vi "Facade.vi"(0 "Data In":T4, 2 "Display State In":T2, 3 "Container State":T3) -> (6 "Data Out":T4, 7 "Display State Out":T2, 8 "Action":T1)   [LabVIEW 2015, in "Vowel.xctl"]
uses:
  Vowel.xctl
  Vowel.Properties.ctl
  <vilib>/_xctls/Container State.ctl
  State.ctl
  <vilib>/_xctls/Action.ctl
  <vilib>/_xctls/XControlSupport.lvlib
panel:
  in  "Level is":enum16{"total power", "per component"}(ring)
  in  "Frequency (Hz)":string
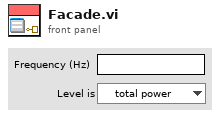
[diagram p1: front panel]
types:
  T1 = typedef "XControlSupport.lvlib/Action.ctl" = cluster{"Data Changed?":bool, "State Changed?":bool, "Action Name":string}
  T2 = typedef "Vowel.xctl/State.ctl" = cluster{"enable menu":bool, "ctls":cluster{"Freq":refnum<vi>, "Phase":refnum<vi>}}
  T3 = typedef "XControlSupport.lvlib/Container State.ctl" = cluster{"Indicator?":bool, "Run Mode?":bool, " Refnum":refnum<vi>}
  T4 = typedef "Vowel.xctl/Vowel.Properties.ctl" = cluster{"Freqs":string, "Set level":enum16{"Total", "Per component"}, "Freq":dbl[], "weights":dbl[]}
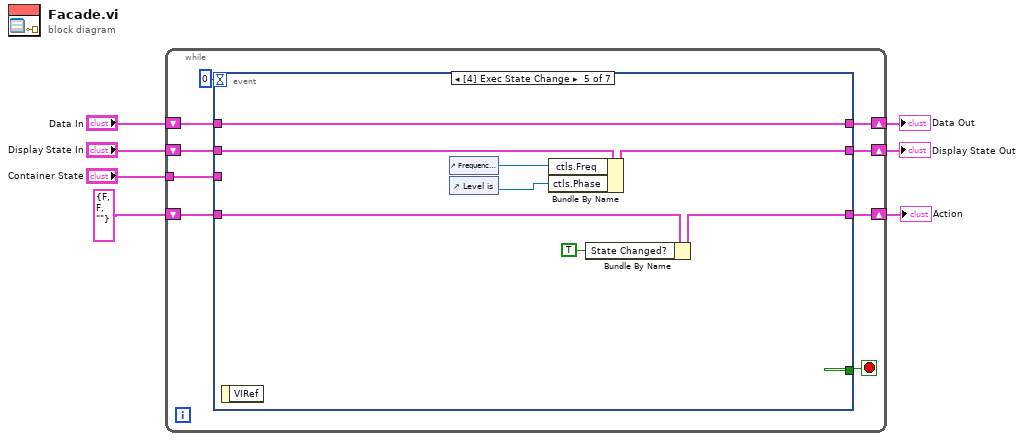
[diagram p0: block diagram]
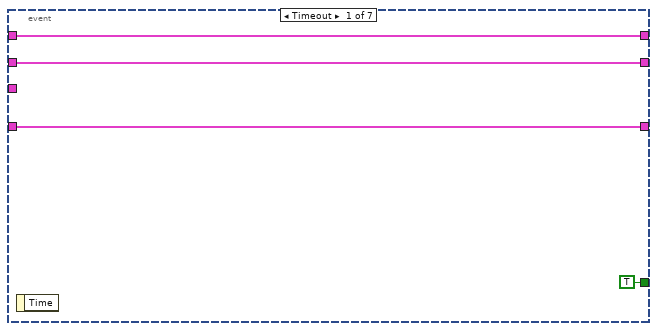
[diagram p2: hidden frame]
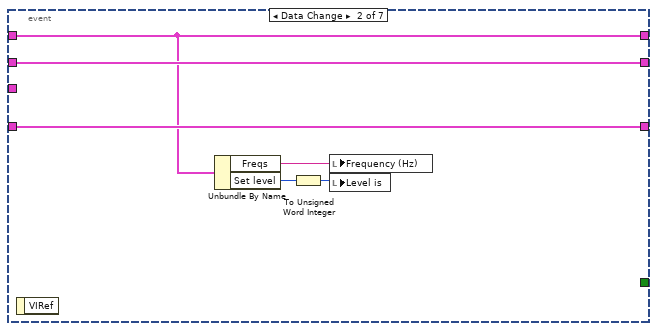
[diagram p3: hidden frame]
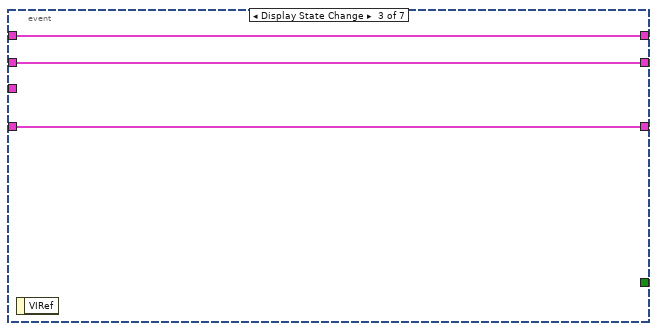
[diagram p4: hidden frame]
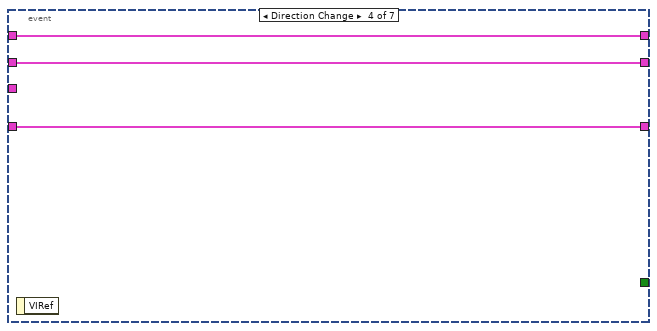
[diagram p5: hidden frame]
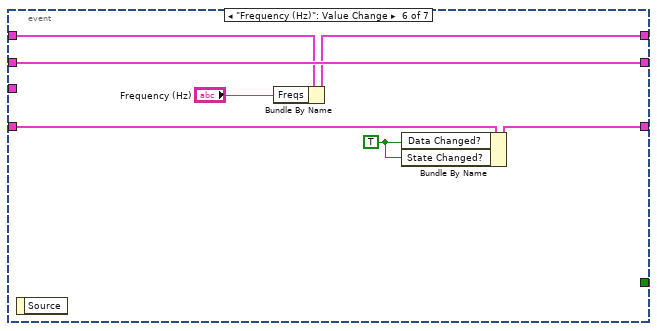
[diagram p6: hidden frame]
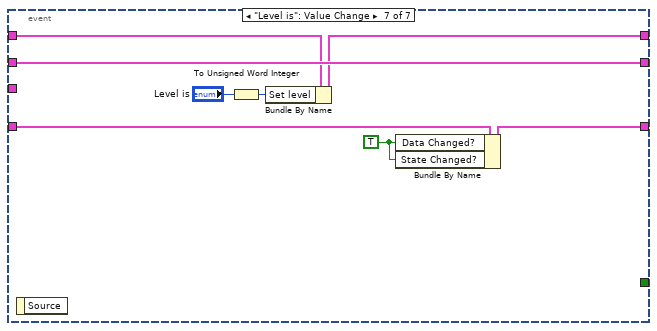
[diagram p7: hidden frame]
diagram:
  n1 = while {
    shift-right: [w15] -> w4
    shift-left: "Display State In" -> [w16]
    tunnel: "Container State" -> [w12]
    shift-right: [w10] -> w7
    shift-left: "Data In" -> [w11]
    shift-right: [w8] -> w2
    shift-left: T1 {"Data Changed?"=FALSE, "State Changed?"=FALSE, "Action Name"=""} ("Action") -> [w9]
    stop <- w14 stop-if-true
    n2 = event shown="[4] Exec State Change" {
      selector: _ -> [_ _ _ _ _ _ _]
      dyn-events: _ -> [_ _ _ _ _ _ _]
      timeout: 0 -> [_ _ _ _ _ _ _]
      tunnel: w16 -> [w18 w26 w27 w32 w40 w47 w55]
      tunnel: [w18 w26 w27 w32 w37 w47 w55] -> w15
      tunnel: [TRUE _ _ _ _ _ _] -> w14
      tunnel: w12 -> [_ _ _ _ _ _ _]
      tunnel: w11 -> [w17 w24 w29 w31 w39 w46 w54]
      tunnel: [w17 w24 w29 w31 w39 w44 w52] -> w10
      tunnel: [w19 w25 w28 w30 w36 w43 w51] -> w8
      tunnel: w9 -> [w19 w25 w28 w30 w38 w45 w53]
      event Timeout {
        n3 = event-data() -> ()  [unwired: 1 in, 1 out]
      }
      event Data Change {
        n4 = event-data() -> ()  [unwired: 1 in, 1 out]
        n5 = Unbundle By Name(w24) -> ("Freqs"=w23:string, "Set level"=w22:enum16{"Total", "Per component"})
        n6 = To Unsigned Word Integer(number=w22) -> (unsigned 16bit integer=w21:u16)
        n7 = local write "Frequency (Hz)"(w23) -> ()
        n8 = local write "Level is"(w21) -> ()
      }
      event Display State Change {
        n9 = event-data() -> ()  [unwired: 1 in, 1 out]
      }
      event Direction Change {
        n10 = event-data() -> ()  [unwired: 1 in, 1 out]
      }
      event Exec State Change {
        n11 = event-data() -> ()  [unwired: 1 in, 1 out]
        n12 = control-ref of="Frequency (Hz)"() -> (w34:refnum<vi>)
        n13 = control-ref of="Level is"() -> (w33:refnum<vi>)
        n14 = Bundle By Name(cluster=w40, "ctls.Freq"=w34, "ctls.Phase"=w33) -> (w37:T2)
        n15 = Bundle By Name(cluster=w38, "State Changed?"=TRUE) -> (w36:T1)
      }
      event "Frequency (Hz)": Value Change {
        w41 = TRUE ("Data Changed?")
        n16 = event-data() -> ()  [unwired: 1 in, 1 out]
        n17 = Bundle By Name(cluster=w46, "Freqs"="Frequency (Hz)") -> (w44:T4)
        n18 = Bundle By Name(cluster=w45, "Data Changed?"=w41, "State Changed?"=w41) -> (w43:T1)
      }
      event "Level is": Value Change {
        w50 = TRUE ("Data Changed?")
        n19 = event-data() -> ()  [unwired: 1 in, 1 out]
        n20 = To Unsigned Word Integer(number="Level is") -> (unsigned 16bit integer=w48:u16)
        n21 = Bundle By Name(cluster=w54, "Set level"=w48) -> (w52:T4)
        n22 = Bundle By Name(cluster=w53, "Data Changed?"=w50, "State Changed?"=w50) -> (w51:T1)
      }
    }
  }
  "Display State Out" <- w4
  "Data Out" <- w7
  "Action" <- w2
